vi "周期设置_总磷总氮.vi"() -> ()   [LabVIEW 2016, in "斯坦道总磷总氮.lvlib"]
uses:
  <vilib>/Utility/miscctls.llb/LVPointTypeDef.ctl
  <vilib>/Utility/config.llb/NI_LVConfig.lvlib
panel:
  in  "运行周期":T1={"运行模式"=enum."维护模式", "质控频次"=enum."关闭", "空白核查时间"=2, "跨度核查时间"=6, "24H周期设置"=[]} {"跨度核查时间" items=["00H", "01H", "02H", "03H", "04H", "05H", "06H", "07H", "08H", "09H", "10H", "11H", "12H", "13H", "14H", "15H", "16H", "17H", "18H", "19H", "20H", "21H", "22H", "23H", "关闭"]; "空白核查时间" items=["00H", "01H", "02H", "03H", "04H", "05H", "06H", "07H", "08H", "09H", "10H", "11H", "12H", "13H", "14H", "15H", "16H", "17H", "18H", "19H", "20H", "21H", "22H", "23H", "关闭"]}
  # "运行模式："
  # "质控频次："
  # "空白核查时间："
  # "跨度核查时间："
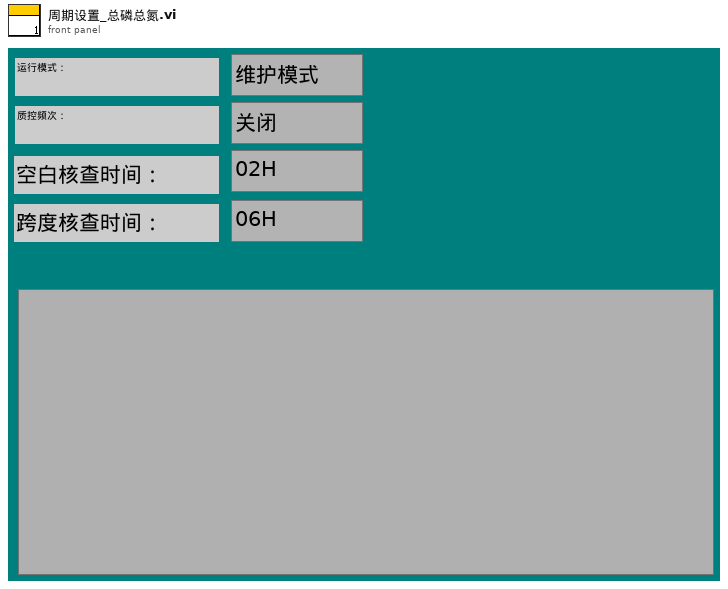
[diagram p1: front panel]
types:
  T1 = cluster{"运行模式":enum16{"维护模式", "常规模式", "应急模式", "质控模式"}, "质控频次":enum16{"关闭", "每天", "星期一", "星期二", "星期三", "星期四", "星期五", "星期六", "星期日"}, "空白核查时间":u16, "跨度核查时间":u16, "24H周期设置":bool[]}
  T2 = typedef "LVPointTypeDef.ctl" = cluster{"Horizontal":i16, "Vertical":i16}
  T3 = enum16{"启动测量", "标样核查", "零点核查", "跨度核查", "空白测试", "平行样测试", "加标回收", "空白校准", "标样校准", "初始化（清洗）", "停止测试", "仪器重启", "校时", "模式设置", "测量间隔设置"}
  T4 = enum16{"关闭", "每天", "星期一", "星期二", "星期三", "星期四", "星期五", "星期六", "星期日"}
  T5 = typedef "LVDateTimeRec.ctl" = cluster{"秒数的小数部分":dbl, "秒":i32, "分":i32, "时":i32, "日":i32, "月":i32, "年":i32, "天数（周）":i32, "天数（年）":i32, "DST":i32}
  T6 = enum32{"Bad", "Idle", "Run top level", "Running"}
  T7 = typedef "NI_LVConfig.lvlib/Config Data RefNum.ctl" = refnum<k1>
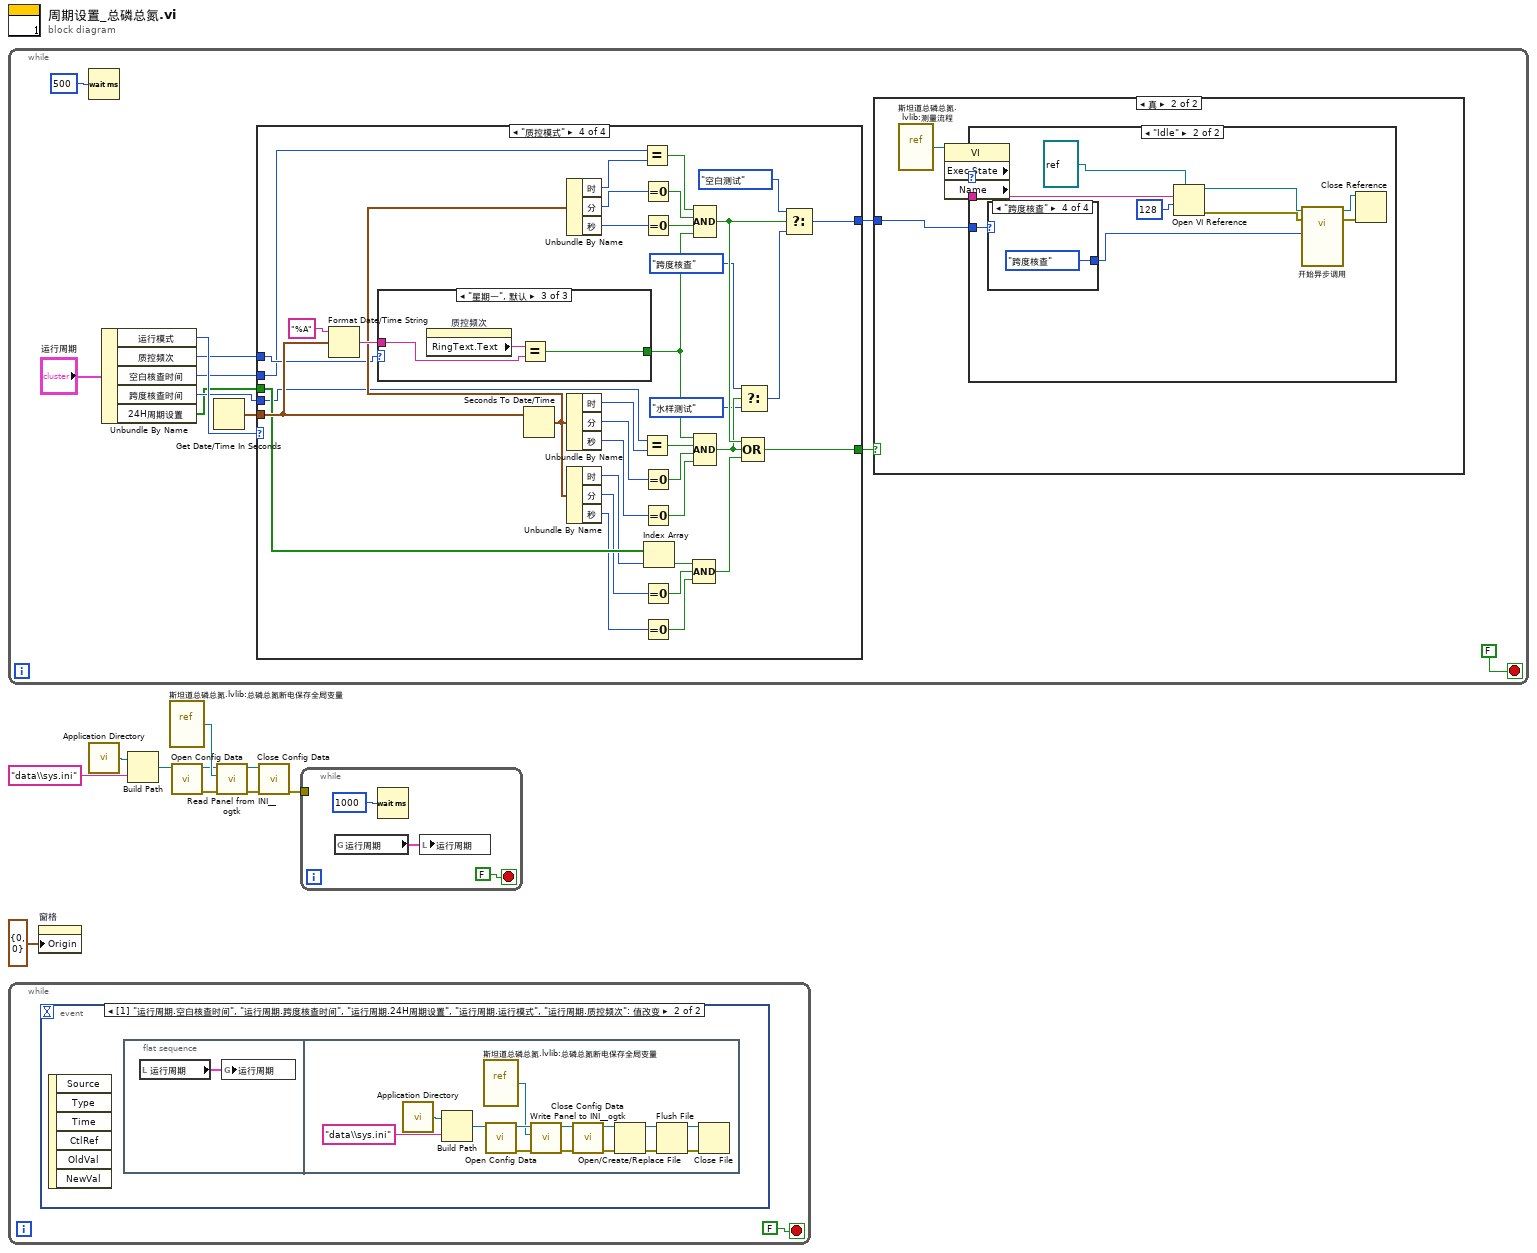
[diagram p0: block diagram]
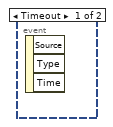
[diagram p2: hidden frame]
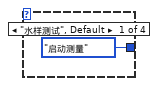
[diagram p5: hidden frame]
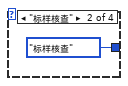
[diagram p6: hidden frame]
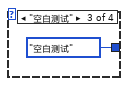
[diagram p7: hidden frame]
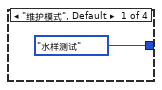
[diagram p8: hidden frame]
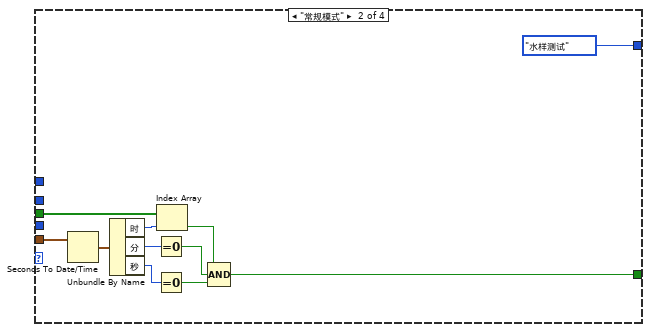
[diagram p9: hidden frame]
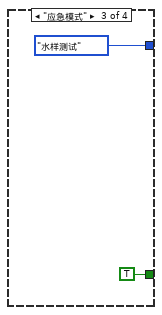
[diagram p10: hidden frame]
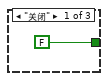
[diagram p11: hidden frame]
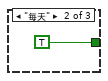
[diagram p12: hidden frame]
diagram:
  n1 = while {
    stop <- FALSE stop-if-true
    n2 = Wait (ms)(milliseconds to wait=u32 500 ("等待时间（毫秒）")) -> ()  [unwired: 1 out]
    n3 = Unbundle By Name("运行周期") -> ("运行模式"=w17:enum16{"维护模式", "常规模式", "应急模式", "质控模式"}, "质控频次"=w16:T4, "空白核查时间"=w15:u16, "跨度核查时间"=w14:u16, "24H周期设置"=w13:bool[])
    n4 = Get Date/Time In Seconds() -> (seconds since 1Jan1904=w21:timestamp)
    n5 = case shown="\"质控模式\"" w17 {
      tunnel: w21 -> [_ w49 _ w88]
      tunnel: w13 -> [_ w46 _ w85]
      tunnel: [_ w40 TRUE w65] -> w12
      tunnel: [enum16{"水样测试", "标样核查", "空白测试", "跨度核查"}."水样测试" ("仪器测试类型") enum16{"水样测试", "标样核查", "空白测试", "跨度核查"}."水样测试" ("仪器测试类型") enum16{"水样测试", "标样核查", "空白测试", "跨度核查"}."水样测试" ("仪器测试类型") w58] -> w11
      tunnel: w16 -> [_ _ _ w55]
      tunnel: w15 -> [_ _ _ w54]
      tunnel: w14 -> [_ _ _ w53]
      frame "维护模式", Default {
      }
      frame "常规模式" {
        n6 = Seconds To Date/Time(time stamp (now)=w49) -> (date time rec=w48:T5)  [unwired: 1 in]
        n7 = Unbundle By Name(w48) -> ("时"=w47:i32, "分"=w45:i32, "秒"=w44:i32)
        n8 = Equal To 0?(x=w45) -> (x = 0?=w42:bool)
        n9 = Equal To 0?(x=w44) -> (x = 0?=w41:bool)
        n10 = Index Array(array=w46, index=w47) -> (element=w43:bool)
        n11 = Compound Arithmetic op=AND ("复合运算")(w43, w42, w41) -> (w40:bool)
      }
      frame "应急模式" {
      }
      frame "质控模式" {
        n12 = Format Date/Time String(time format string (%c)="%A" ("时间格式字符串(%c)"), seconds (now)=w88) -> (date/time string=w86:string)  [unwired: 1 in]
        n13 = case shown="\"星期一\", 默认" w55 {
          tunnel: w86 -> [_ _ w92]
          tunnel: [FALSE TRUE w91] -> w56
          frame "关闭" {
          }
          frame "每天" {
          }
          frame "星期一", Default {
            n14 = property on="质控频次" class="Enum (严格)"() -> ("RingText.Text"=w93:string)  [unwired: 2 in, 2 out]
            n15 = Equal?(x=w93, y=w92) -> (x = y?=w91:bool)
          }
        }
        n16 = Seconds To Date/Time(time stamp (now)=w88) -> (date time rec=w69:T5)  [unwired: 1 in]
        n17 = Unbundle By Name(w69) -> ("时"=w78:i32, "分"=w77:i32, "秒"=w76:i32)
        n18 = Unbundle By Name(w69) -> ("时"=w70:i32, "分"=w71:i32, "秒"=w72:i32)
        n19 = Unbundle By Name(w69) -> ("时"=w84:i32, "分"=w82:i32, "秒"=w80:i32)
        n20 = Equal?(x=w54, y=w78) -> (x = y?=w75:bool)
        n21 = Equal?(x=w53, y=w70) -> (x = y?=w68:bool)
        n22 = Equal To 0?(x=w77) -> (x = 0?=w74:bool)
        n23 = Equal To 0?(x=w76) -> (x = 0?=w73:bool)
        n24 = Equal To 0?(x=w71) -> (x = 0?=w67:bool)
        n25 = Equal To 0?(x=w72) -> (x = 0?=w66:bool)
        n26 = Equal To 0?(x=w82) -> (x = 0?=w81:bool)
        n27 = Equal To 0?(x=w80) -> (x = 0?=w79:bool)
        n28 = Index Array(array=w85, index=w84) -> (element=w83:bool)
        n29 = Compound Arithmetic op=AND ("复合运算")(w83, w81, w79) -> (w57:bool)
        n30 = Compound Arithmetic op=AND ("复合运算")(w75, w74, w73, w56) -> (w64:bool)
        n31 = Compound Arithmetic op=AND ("复合运算")(w56, w68, w67, w66) -> (w62:bool)
        n32 = Select(t=enum16{"水样测试", "标样核查", "空白测试", "跨度核查"}."跨度核查" ("仪器测试类型"), s=w62, f=enum16{"水样测试", "标样核查", "空白测试", "跨度核查"}."水样测试" ("仪器测试类型")) -> (s? t:f=w60:enum16{"水样测试", "标样核查", "空白测试", "跨度核查"})
        n33 = Compound Arithmetic op=OR ("复合运算")(w64, w62, w57) -> (w65:bool)
        n34 = Select(t=enum16{"水样测试", "标样核查", "空白测试", "跨度核查"}."空白测试" ("仪器测试类型"), s=w64, f=w60) -> (s? t:f=w58:enum16{"水样测试", "标样核查", "空白测试", "跨度核查"})
      }
    }
    n35 = case shown="真" w12 {
      tunnel: w11 -> [_ w23]
      frame False {
      }
      frame True {
        n36 = vi-ref "斯坦道总磷总氮.lvlib:测量流程.vi"() -> (w24:refnum<vi>)
        n37 = property class="VI"(reference=w24) -> ("Exec.State"=w22:T6, "Name"=w25:string)  [unwired: 1 in, 2 out]
        n38 = case shown="\"Idle\"" w22 {
          tunnel: w25 -> [_ w30]
          tunnel: w23 -> [_ w28]
          frame "Bad", Default {
          }
          frame "Idle" {
            n39 = case shown="\"跨度核查\"" w28 {
              tunnel: [T3."启动测量" ("控制命令") T3."标样核查" ("控制命令") T3."空白测试" ("控制命令") T3."跨度核查" ("控制命令")] -> w26
              frame "水样测试", Default {
              }
              frame "标样核查" {
              }
              frame "空白测试" {
              }
              frame "跨度核查" {
              }
            }
            n40 = Open VI Reference(type specifier VI Refnum (for type only)=refnum<vi> refnum, vi path=w30, options=128 ("选项")) -> (vi reference=w31:refnum<vi>, error out=w32:errorcluster)  [unwired: 3 in]
            n41 = call-by-ref "开始异步调用"(reference=w31, error in=w32, "控制命令"=w26) -> (reference out=w33:refnum<vi>, error out=w34:errorcluster)  [unwired: 11 in]
            n42 = Close Reference(reference=w33, error in (no error)=w34) -> ()  [unwired: 1 out]
          }
        }
      }
    }
  }
  n43 = while {
    stop <- FALSE stop-if-true
    n44 = event shown="[1] \"运行周期.空白核查时间\", \"运行周期.跨度核查时间\", \"运行周期.24H周期设置\", \"运行周期.运行模式\", \"运行周期.质控频次\": 值改变" {
      selector: _ -> [_ _]
      dyn-events: _ -> [_ _]
      timeout: _ -> [_ _]
      event Timeout {
        n45 = event-data() -> ()  [unwired: 1 in, 3 out]
      }
      event "运行周期.空白核查时间", "运行周期.跨度核查时间", "运行周期.24H周期设置", "运行周期.运行模式", "运行周期.质控频次": Value Change {
        n46 = event-data() -> ()  [unwired: 1 in, 6 out]
        n47 = flat-sequence {
          frame #0 {
            n48 = local read "运行周期"() -> (w95:T1)
            n49 = global write "总磷总氮断电保存全局变量.vi" "运行周期"(w95) -> ()
          }
          frame #1 {
            n50 = call <vilib>:"Application Directory.vi"() -> ("Application Directory"=w109:path)
            n51 = Build Path(base path=w109, name or relative path="data\\sys.ini" ("名称或相对路径")) -> (appended path=w107:path)
            n52 = vi-ref "斯坦道总磷总氮.lvlib:总磷总氮断电保存全局变量.vi"() -> (w105:refnum<vi>)
            n53 = call <vilib>:"Open Config Data.vi"("configuration file path"=w107) -> ("error out"=w103:errorcluster, "refnum"=w106:T7)  [unwired: 8 in, 1 out]
            n54 = call <userlib>:"Write Panel to INI__ogtk.vi"("error in (no error)"=w103, "VI ref"=w105, "refnum"=w106) -> ("error out"=w102:errorcluster, "refnum out"=w104:T7)  [unwired: 7 in]
            n55 = call <vilib>:"Close Config Data.vi"("error in (no error)"=w102, "refnum"=w104) -> ("error out"=w97:errorcluster, "file path"=w96:path)  [unwired: 8 in]
            n56 = Open/Create/Replace File(file path (use dialog)=w96, error in=w97) -> (refnum out=w100:refnum<file>, error out=w101:errorcluster)  [unwired: 4 in, 1 out]
            n57 = Flush File(refnum=w100, error in=w101) -> (refnum out=w99:refnum<file>, error out=w98:errorcluster)
            n58 = Close File(refnum=w99, error in=w98) -> ()  [unwired: 2 out]
          }
        }
      }
    }
  }
  n59 = property on="窗格" class="Pane"("Origin"=T2 {"Horizontal"=0, "Vertical"=0} ("原点")) -> ()  [unwired: 2 in, 2 out]
  n60 = call <vilib>:"Application Directory.vi"() -> ("Application Directory"=w3:path)
  n61 = Build Path(base path=w3, name or relative path="data\\sys.ini" ("名称或相对路径")) -> (appended path=w5:path)
  n62 = vi-ref "斯坦道总磷总氮.lvlib:总磷总氮断电保存全局变量.vi"() -> (w7:refnum<vi>)
  n63 = call <vilib>:"Open Config Data.vi"("configuration file path"=w5) -> ("error out"=w9:errorcluster, "refnum"=w6:T7)  [unwired: 8 in, 1 out]
  n64 = call <userlib>:"Read Panel from INI__ogtk.vi"("error in (no error)"=w9, "VI ref"=w7, "refnum"=w6) -> ("error out"=w10:errorcluster, "refnum out"=w8:T7)  [unwired: 7 in]
  n65 = call <vilib>:"Close Config Data.vi"("error in (no error)"=w10, "refnum"=w8) -> ("error out"=w2:errorcluster)  [unwired: 8 in, 1 out]
  n66 = while {
    tunnel: w2 -> [_]
    stop <- FALSE stop-if-true
    n67 = global read "总磷总氮断电保存全局变量.vi" "运行周期"() -> (w110:T1)
    n68 = Wait (ms)(milliseconds to wait=u32 1000 ("等待时间（毫秒）")) -> ()  [unwired: 1 out]
    n69 = local write "运行周期"(w110) -> ()
  }
